vi "Keysight34461a.vi"(10 "Measurement Function (10: Voltage DC)":i32(ring)=10 items=["Continuity", "Current AC", "Current DC", "Diode", "Frequency", "Resistance 4-wire", "Period", "Resistance 2-wire", "Temperature", "Voltage AC", "Voltage DC", "Voltage DC Ratio", "Capacitance"], 11 "VISA resource name":refnum<visa-resource-name>) -> (3 "Display":string)   [LabVIEW 2024, in "Keysight_34461a.lvlib"]
doc: "This template is for the Queued Message Handler design pattern.\n\nThe Event Handling Loop generates messages based on user interface actions.\n\nThe Message Handling Loop processes messages generated by the Event Handling Loop, or by other messages. The messages are string values, so new messages can be added easily to the Message Cases case structure in the Message Handling Loop. Each message cluster can also provide an optional value for Message Data, which is a variant that can be converted to whatever message-specific data is required."
uses:
  Keysight_34461a.lvlib
  Settings/support/DMM_CONFIG.ctl
  controls/UI Data.ctl
  support/Message Queue/Enqueue Message (Single).vi
  <instrlib>/Agilent 3446X Series/Public/Data/Read (Single Point).vi
  <vilib>/Utility/error.llb/Error Cluster From Error Code.vi
  <vilib>/ErrorRing/Error Ring.xnode
  support/Message Queue/Message Queue.lvlib
  support/User Event - Stop/User Event - Stop.lvlib
  <instrlib>/Agilent 3446X Series/Agilent 3446X Series.lvlib
  Settings/Setting_Screen.lvlib
  Launcher/Launcher_DTU.lvlib
panel:
  in  "Read":bool
  in  "DMM_CONFIG":T1 {"CONFIG PARAMETER" items=["VOLTAGE", "CURRENT", "RESISTANCE", "POWER"]}
  in  "Config":string
  in  "DUT":string
  out "queue name 2":string
  out "queue name":string
  in  "Exit":bool
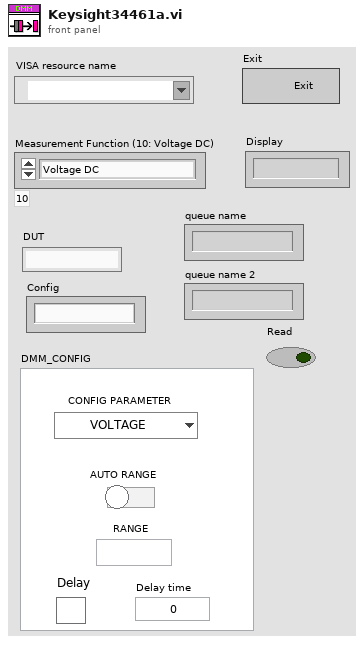
[diagram p1: front panel]
types:
  T1 = typedef "Setting_Screen.lvlib/DMM_CONFIG.ctl" = cluster{"CONFIG PARAMETER":u16, "AUTO RANGE":bool, "RANGE":string, "Delay":bool, "Delay time":dbl}
  T2 = typedef "Keysight_34461a.lvlib/UI Data.ctl" = cluster{"Boolean <Replace Me>":bool, "Display":string, "Numeric <Replace Me>":dbl, "Data Display Ref":refnum<vi>, "Exit Button Ref":refnum<vi>, "VISA resource name":refnum<visa-resource-name>, "notifier out":refnum<notifier>, "Config":string, "DUT":string, "Keysight_34461a_Q":refnum<queue>, "Config 2":string, "Count":u32}
  T3 = typedef "Keysight_34461a.lvlib/Message Queue.lvlib/All Message Queues.ctl" = cluster{"UI":refnum<queue>, "QSM":refnum<queue>}
  T4 = cluster{"Message":string, "Message Data":variant}
  T5 = enum16{"Read", "Write", "All_sections", "All_values", "Remove key&section"}
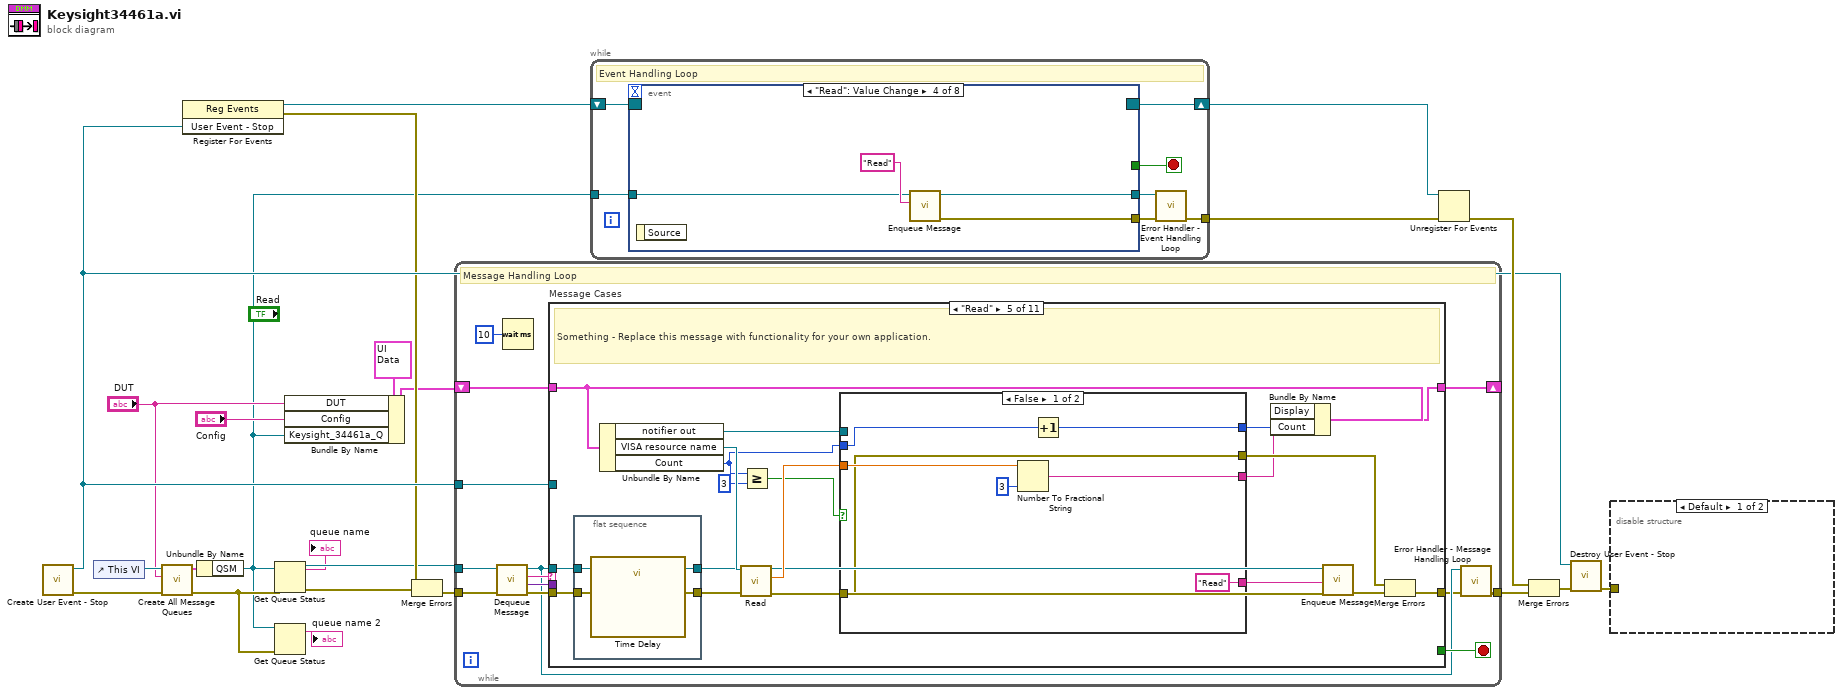
[diagram p0: block diagram]
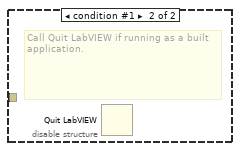
[diagram p2: hidden frame]
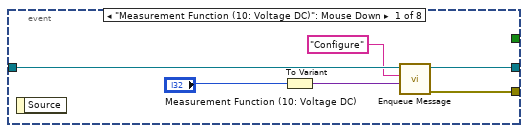
[diagram p3: hidden frame]
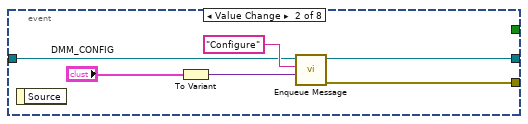
[diagram p4: hidden frame]
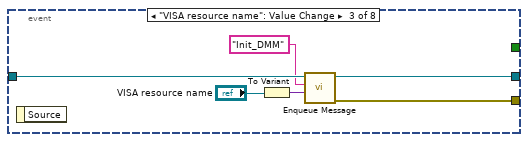
[diagram p5: hidden frame]
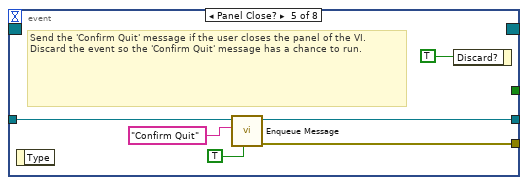
[diagram p6: hidden frame]
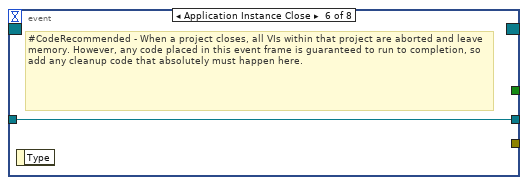
[diagram p7: hidden frame]
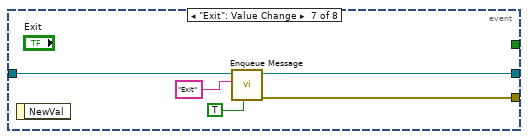
[diagram p8: hidden frame]
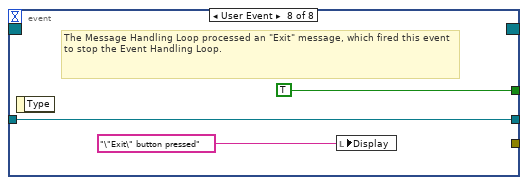
[diagram p9: hidden frame]
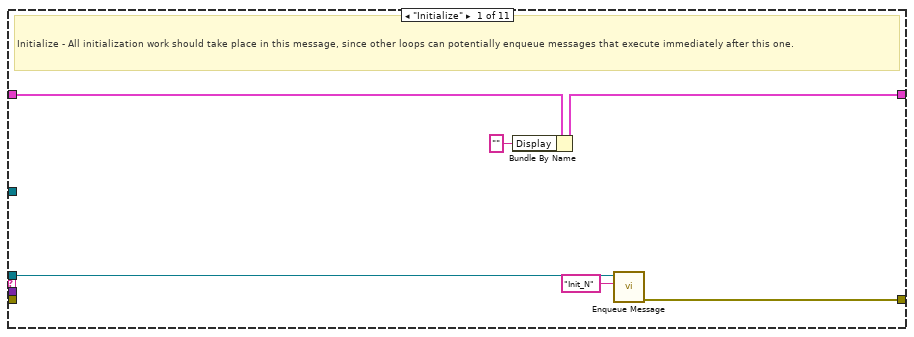
[diagram p10: hidden frame]
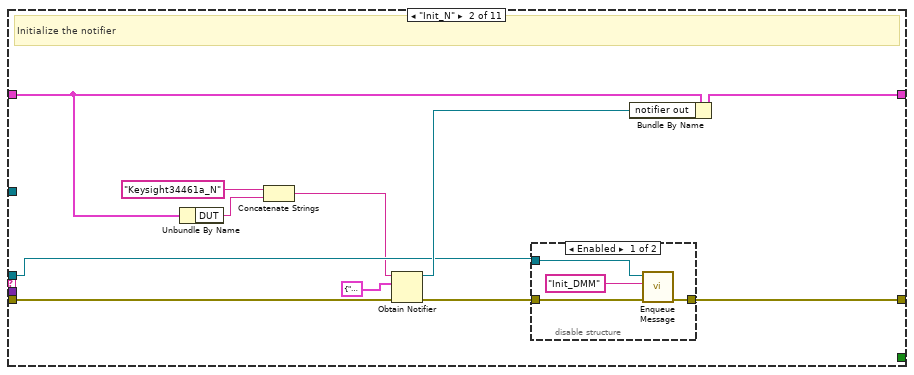
[diagram p11: hidden frame]
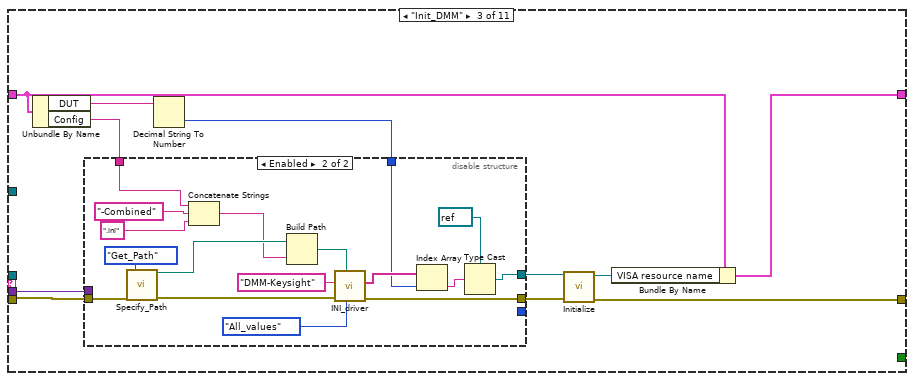
[diagram p13: hidden frame]
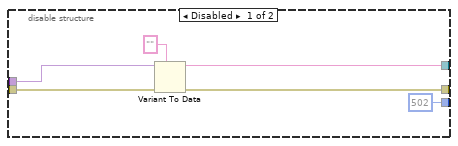
[diagram p14: hidden frame]
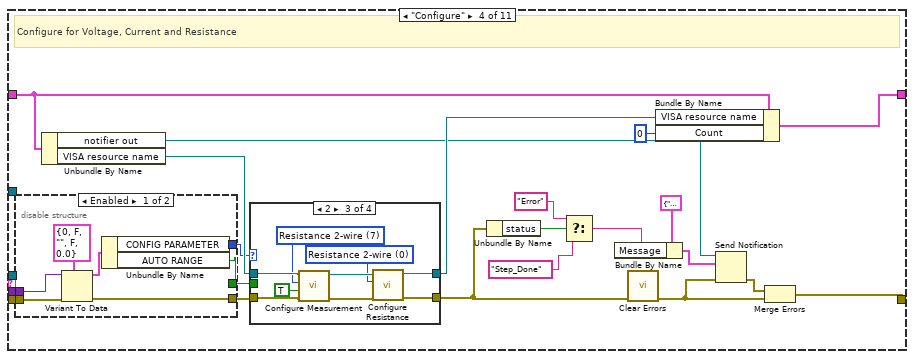
[diagram p15: hidden frame]
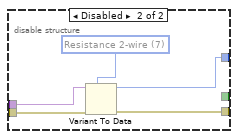
[diagram p16: hidden frame]
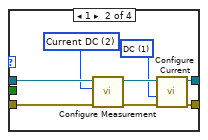
[diagram p18: hidden frame]
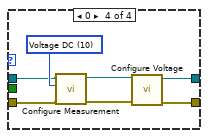
[diagram p19: hidden frame]
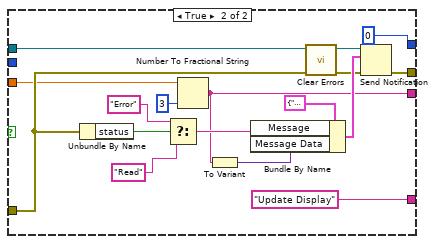
[diagram p20: hidden frame]
diagram:
  n1 = call "Create User Event - Stop.vi"() -> ("error out"=w21:errorcluster, "User Event - Stop"=w14:refnum<user-event>)  [unwired: 10 in]
  n2 = control-ref of="This VI"() -> (w5:refnum<vi>)
  n3 = call "Create All Message Queues.vi"("error in (no error)"=w21, "DUT"="DUT", "This VI"=w5) -> ("error out"=w8:errorcluster, "Message Queues out"=w23:T3)  [unwired: 7 in]
  n4 = register-events(w14) -> (reference out=w15:refnum<event-registration>, error out=w12:errorcluster)  [unwired: 2 in]
  n5 = Unbundle By Name(w23) -> ("QSM"=w1:refnum<queue>)
  n6 = Get Queue Status(queue=w1, error in (no error)=w8) -> (queue out=w10:refnum<queue>, queue name=→"queue name":string, error out=w11:errorcluster)  [unwired: 1 in, 5 out]
  n7 = Get Queue Status(queue=w1, error in (no error)=w8) -> (queue name=→"queue name 2":string)  [unwired: 1 in, 7 out]
  n8 = Bundle By Name(cluster=T2 {"Boolean <Replace Me>"=FALSE, "Display"="", "Numeric <Replace Me>"=0.0, "Data Display Ref"=refnum, "Exit Button Ref"=refnum, "VISA resource name"="", "notifier out"=refnum, "Config"="", "DUT"="", "Keysight_34461a_Q"=refnum, "Config 2"="", "Count"=0} ("Data Cluster"), "DUT"="DUT", "Config"="Config", "Keysight_34461a_Q"=w1) -> (w4:T2)
  n9 = Merge Errors(w12, w11) -> (w13:errorcluster)
  n10 = while {
    tunnel: w10 -> [w28]
    shift-right: [w35] -> _
    shift-left: w4 -> [w36]
    tunnel: w14 -> [w33]
    tunnel: w13 -> [w32]
    tunnel: [w26] -> w22
    stop <- w34 stop-if-true
    # "Message Handling Loop"
    n11 = call "Dequeue Message.vi"("error in (no error)"=w32, "Message Queue"=w28) -> ("error out"=w31:errorcluster, "Message Data"=w29:variant, "Message"=w30:string, "dup Message Queue"=w27:refnum<queue>)  [unwired: 6 in]
    n12 = Wait (ms)(milliseconds to wait=u32 10) -> ()  [unwired: 1 out]
    n13 = case "Message Cases" shown="\"Read\"" w30 {
      selector: w30 -> [_ _ _ _ _ _ _ _ _ _ w232]
      tunnel: w27 -> [w39 w46 _ _ w157 _ _ _ w215 w231 _]
      tunnel: w31 -> [_ w51 w65 w113 w159 w199 w205 w207 w210 w222 _]
      tunnel: [w42 w47 w69 w98 w165 w199 w200 w207 w216 w228 w233] -> w25
      tunnel: w36 -> [w41 w44 w62 w110 w167 w198 w204 w206 w212 w221 w234]
      tunnel: [w40 w50 w67 w107 w166 w198 w204 w206 w212 w221 w234] -> w35
      tunnel: [_ _ _ _ _ _ _ _ _ TRUE _] -> w34
      tunnel: w29 -> [_ _ w64 w112 _ _ w203 _ _ w223 _]
      tunnel: w33 -> [_ _ _ _ _ _ _ _ _ w227 _]
      frame "Initialize" {
        # "Initialize - All initialization work should take place in this message, since other loops can potentially enqueue messages that execute immediately after this one."
        n14 = Bundle By Name(cluster=w41, "Display"="") -> (w40:T2)
        n15 = call-poly "Enqueue Message.vi"("Message"="Init_N", "Message Queue"=w39) -> ("error out"=w42:errorcluster)  [unwired: 8 in, 1 out]
      }
      frame "Init_N" {
        # "Initialize the notifier"
        n16 = Unbundle By Name(w44) -> ("DUT"=w43:string)
        n17 = Concatenate Strings("Keysight34461a_N" ("String"), w43) -> (w45:string)
        n18 = Obtain Notifier(name (unnamed)=w45, notification data type=T4 {"Message"="", "Message Data"=variant} ("notification"), error in (no error)=w51) -> (notifier out=w49:refnum<notifier>, error out=w48:errorcluster)  [unwired: 1 in, 1 out]
        n19 = disable-structure shown="Enabled" {
          disable-tunnel: w48 -> [w56 w58]
          disable-tunnel: [w55 w58] -> w47
          disable-tunnel: w46 -> [w54 _]
          frame Enabled {
            n20 = call-poly "Enqueue Message.vi"("error in (no error)"=w56, "Message"="Init_DMM", "Message Queue"=w54) -> ("error out"=w55:errorcluster)  [unwired: 7 in, 1 out]
          }
          frame Disabled {
          }
        }
        n21 = Bundle By Name(cluster=w44, "notifier out"=w49) -> (w50:T2)
      }
      frame "Init_DMM" {
        n22 = Unbundle By Name(w62) -> ("DUT"=w60:string, "Config"=w63:string)
        n23 = Decimal String To Number(string=w60) -> (number=w59:i32)  [unwired: 2 in, 1 out]
        n24 = disable-structure shown="Enabled" {
          disable-tunnel: w65 -> [w75 w85]
          disable-tunnel: [w74 w84] -> w66
          disable-tunnel: w64 -> [w73 _]
          disable-tunnel: [w72 w79] -> w61
          disable-tunnel: [u16 502 _] -> _
          disable-tunnel: w63 -> [_ w80]
          disable-tunnel: w59 -> [_ w76]
          frame Disabled {
            n25 = Variant To Data(error in=w75, type="", Variant=w73) -> (data=w72:string, error out=w74:errorcluster)
          }
          frame Enabled {
            n26 = call "Specify_Path.vi"("Path_Enum"=enum16{"Find_Path", "Get_Path"}."Get_Path", "error in (no error)"=w85) -> ("Configurations"=w91:path, "error out"=w88:errorcluster)  [unwired: 6 in, 6 out]
            n27 = Concatenate Strings(w80, "-Combined" ("string"), ".ini" ("string")) -> (w81:string)
            n28 = Build Path(base path=w91, name or relative path=w81) -> (appended path=w90:path)
            n29 = call "INI_driver.vi"("Enum"=T5."All_values", "instrument file path"=w90, "error in (no error)"=w88, "Section"="DMM-Keysight") -> ("error out"=w84:errorcluster, "Values out"=w86:string[])  [unwired: 4 in, 2 out]
            n30 = Index Array(array=w86, index=w76) -> (element=w78:string)
            n31 = Type Cast(type=refnum<visa-resource-name> refnum ("VISA resource name 2"), x=w78) -> (*(type *) &x=w79:refnum<visa-resource-name>)
          }
        }
        n32 = call <instrlib>:"Initialize.vi"("error in (no error)"=w66, "VISA resource name"=w61) -> ("error out"=w69:errorcluster, "VISA resource name out"=w68:refnum<visa-resource-name>)  [unwired: 8 in]
        n33 = Bundle By Name(cluster=w62, "VISA resource name"=w68) -> (w67:T2)
      }
      frame "Configure" {
        # "Configure for Voltage, Current and Resistance"
        n34 = disable-structure shown="Enabled" {
          disable-tunnel: w113 -> [w120 w125]
          disable-tunnel: w112 -> [w119 w122]
          disable-tunnel: [w118 w124] -> w111
          disable-tunnel: [w116 w121] -> w108
          disable-tunnel: [w114 _] -> w94
          frame Enabled {
            n35 = Variant To Data(error in=w120, type=T1 {"CONFIG PARAMETER"=0, "AUTO RANGE"=FALSE, "RANGE"="", "Delay"=FALSE, "Delay time"=0.0} ("DMM_CONFIG"), Variant=w119) -> (data=w115:T1, error out=w118:errorcluster)
            n36 = Unbundle By Name(w115) -> ("CONFIG PARAMETER"=w116:u16, "AUTO RANGE"=w114:bool)
          }
          frame Disabled {
            w123 = 7 items=["Continuity", "Current AC", "Current DC", "Diode", "Frequency", "Resistance 4-wire", "Period", "Resistance 2-wire", "Temperature", "Voltage AC", "Voltage DC", "Voltage DC Ratio", "Capacitance"] ("Measurement Function (10: Voltage DC)")
            n37 = Variant To Data(error in=w125, type=w123, Variant=w122) -> (data=w121:i32, error out=w124:errorcluster)
          }
        }
        n38 = Unbundle By Name(w110) -> ("notifier out"=w100:refnum<notifier>, "VISA resource name"=w109:refnum<visa-resource-name>)
        n39 = case shown="2" w108 {
          tunnel: w111 -> [w127 w133 w142 w146]
          tunnel: [w127 w135 w144 w151] -> w97
          tunnel: w109 -> [w126 w132 w140 w148]
          tunnel: [w126 w134 w143 w150] -> w106
          tunnel: w94 -> [_ _ _ _]
          frame Default {
          }
          frame 1 {
            w128 = 1 items=["AC", "DC"] ("Current Type (0: AC)")
            w129 = 2 items=["Continuity", "Current AC", "Current DC", "Diode", "Frequency", "Resistance 4-wire", "Period", "Resistance 2-wire", "Temperature", "Voltage AC", "Voltage DC", "Voltage DC Ratio", "Capacitance"] ("Measurement Function (10: Voltage DC)")
            n40 = call <instrlib>:"Configure Measurement.vi"("error in (no error)"=w133, "Measurement Function (10: Voltage DC)"=w129, "VISA resource name"=w132) -> ("error out"=w131:errorcluster, "VISA resource name out"=w130:refnum<visa-resource-name>)  [unwired: 7 in]
            n41 = call <instrlib>:"Configure Current.vi"("error in (no error)"=w131, "Current Type (0: AC)"=w128, "VISA resource name"=w130) -> ("error out"=w135:errorcluster, "VISA resource name out"=w134:refnum<visa-resource-name>)  [unwired: 7 in]
          }
          frame 2 {
            w137 = 0 items=["Resistance 2-wire", "Resistance 4-wire"] ("Resistance Type (0: Resistance 2-wire)")
            w138 = 7 items=["Continuity", "Current AC", "Current DC", "Diode", "Frequency", "Resistance 4-wire", "Period", "Resistance 2-wire", "Temperature", "Voltage AC", "Voltage DC", "Voltage DC Ratio", "Capacitance"] ("Measurement Function (10: Voltage DC)")
            n42 = call <instrlib>:"Configure Measurement.vi"("error in (no error)"=w142, "Auto Range (T: Enable)"=TRUE, "Measurement Function (10: Voltage DC)"=w138, "VISA resource name"=w140) -> ("error out"=w141:errorcluster, "VISA resource name out"=w139:refnum<visa-resource-name>)  [unwired: 6 in]
            n43 = call <instrlib>:"Configure Resistance.vi"("error in (no error)"=w141, "Resistance Type (0: Resistance 2-wire)"=w137, "VISA resource name"=w139) -> ("error out"=w144:errorcluster, "VISA resource name out"=w143:refnum<visa-resource-name>)  [unwired: 7 in]
          }
          frame 0 {
            w149 = 10 items=["Continuity", "Current AC", "Current DC", "Diode", "Frequency", "Resistance 4-wire", "Period", "Resistance 2-wire", "Temperature", "Voltage AC", "Voltage DC", "Voltage DC Ratio", "Capacitance"] ("Measurement Function (10: Voltage DC)")
            n44 = call <instrlib>:"Configure Measurement.vi"("error in (no error)"=w146, "Measurement Function (10: Voltage DC)"=w149, "VISA resource name"=w148) -> ("error out"=w145:errorcluster, "VISA resource name out"=w147:refnum<visa-resource-name>)  [unwired: 7 in]
            n45 = call <instrlib>:"Configure Voltage.vi"("error in (no error)"=w145, "VISA resource name"=w147) -> ("error out"=w151:errorcluster, "VISA resource name out"=w150:refnum<visa-resource-name>)  [unwired: 8 in]
          }
        }
        n46 = Unbundle By Name(w97) -> ("status"=w105:bool)
        n47 = Select(t="Error" ("f"), s=w105, f="Step_Done" ("Message")) -> (s? t:f=w102:string)
        n48 = Bundle By Name(cluster=T4 {"Message"="", "Message Data"=variant} ("notification"), "Message"=w102) -> (w101:T4)
        n49 = call <vilib>:"Clear Errors.vi"("error in (no error)"=w97) -> ("error out"=w95:errorcluster)  [unwired: 5 in, 1 out]
        n50 = Bundle By Name(cluster=w110, "VISA resource name"=w106, "Count"=u32 0) -> (w107:T2)
        n51 = Send Notification(notification=w101, notifier=w100, error in (no error)=w95) -> (error out=w96:errorcluster)  [unwired: 1 out]
        n52 = Merge Errors(w96, w95) -> (w98:errorcluster)
      }
      frame "Read" {
        # "Something - Replace this message with functionality for your own application."
        n53 = flat-sequence {
          tunnel: w159 -> [w196]
          tunnel: [w194] -> w158
          tunnel: w157 -> [w195]
          tunnel: [w195] -> w156
          frame #0 {
            n54 = call "Time Delay"("error in (no error)"=w196) -> ("error out"=w194:errorcluster)  [unwired: 10 in]
          }
        }
        n55 = Unbundle By Name(w167) -> ("notifier out"=w163:refnum<notifier>, "VISA resource name"=w168:refnum<visa-resource-name>, "Count"=w152:u32)
        n56 = call-poly <instrlib>:"Read.vi"("error in (no error)"=w158, "VISA resource name"=w168) -> ("error out"=w162:errorcluster, "Measurement"=w161:dbl)  [unwired: 7 in, 1 out]
        n57 = Greater Or Equal?(x=w152, y=u32 3) -> (x >= y?=w154:bool)
        n58 = case shown="False" w154 {
          tunnel: ["Read" ("Message") "Update Display" ("Message")] -> w169
          tunnel: [w173 w186] -> w164
          tunnel: w163 -> [_ w185]
          tunnel: w162 -> [w173 w184]
          tunnel: w161 -> [w176 w182]
          tunnel: [w174 w180] -> w160
          tunnel: [w171 u32 0 ("Count")] -> w153
          tunnel: w152 -> [w172 _]
          frame False {
            n59 = Number To Fractional String(number=w176, precision (6)=i16 3) -> (F-format string=w174:string)  [unwired: 2 in]
            n60 = Increment(x=w172) -> (x+1=w171:u32)
          }
          frame True {
            n61 = Unbundle By Name(w184) -> ("status"=w192:bool)
            n62 = Select(t="Error" ("f"), s=w192, f="Read" ("Message")) -> (s? t:f=w188:string)
            n63 = Number To Fractional String(number=w182, precision (6)=i16 3) -> (F-format string=w180:string)  [unwired: 2 in]
            n64 = To Variant(anything=w180) -> (Variant=w181:variant)
            n65 = Bundle By Name(cluster=T4 {"Message"="", "Message Data"=variant} ("notification"), "Message"=w188, "Message Data"=w181) -> (w187:T4)
            n66 = call <vilib>:"Clear Errors.vi"("error in (no error)"=w184) -> ("error out"=w183:errorcluster)  [unwired: 5 in, 1 out]
            n67 = Send Notification(notification=w187, notifier=w185, error in (no error)=w183) -> (error out=w186:errorcluster)  [unwired: 1 out]
          }
        }
        n68 = Bundle By Name(cluster=w167, "Display"=w160, "Count"=w153) -> (w166:T2)
        n69 = call-poly "Enqueue Message.vi"("error in (no error)"=w162, "Message"=w169, "Message Queue"=w156) -> ("error out"=w170:errorcluster)  [unwired: 7 in, 1 out]
        n70 = Merge Errors(w164, w170) -> (w165:errorcluster)
      }
      frame "Update Display" {
        # "Update Display - Convert the message data to a string to display in the Data Display indicator."
        n71 = Unbundle By Name(w198) -> ("Display"=→"Display":string)
      }
      frame "Error" {
        # "Error - Display an error dialog. This message is sent by the \"Error Handler\" VIs at the end of other loops in this application."
        n72 = Variant To Data(error in=w205, type=errorcluster {"status"=FALSE, "code"=0, "source"=""} ("error constant"), Variant=w203) -> (data=w201:errorcluster, error out=w200:errorcluster)
        n73 = call <vilib>:"Simple Error Handler.vi"("error in (no error)"=w201) -> ()  [unwired: 4 in, 5 out]
      }
      frame "Reset" {
      }
      frame "Confirm Quit" {
        # "Confirm Quit - Message that can confirm whether or not the user wants to exit the application."
        n74 = Unbundle By Name(w212) -> ("notifier out"=w211:refnum<notifier>)
        n75 = Release Notifier(notifier=w211, force destroy? (F)=TRUE, error in (no error)=w210) -> (error out=w209:errorcluster)  [unwired: 2 out]
        n76 = call-poly "Enqueue Message.vi"("Priority Message? (F)"=TRUE, "error in (no error)"=w209, "Message"="Exit", "Message Queue"=w215) -> ("error out"=w216:errorcluster)  [unwired: 6 in, 1 out]
      }
      frame "Exit" {
        # "Stop the VI"
        # "Release the message queue reference"
        # "Exit - Exit the application."
        n77 = Unbundle By Name(w221) -> ("VISA resource name"=w220:refnum<visa-resource-name>)
        n78 = Variant To Data(type=errorcluster {"status"=FALSE, "code"=0, "source"=""} ("error constant"), Variant=w223) -> (data=w224:errorcluster)  [unwired: 1 in, 1 out]
        n79 = call <vilib>:"Simple Error Handler.vi"("error in (no error)"=w224) -> ()  [unwired: 4 in, 5 out]
        n80 = call <instrlib>:"Close.vi"("error in (no error)"=w222, "VISA resource name"=w220) -> ("error out"=w218:errorcluster)  [unwired: 9 in]
        n81 = call "Fire User Event - Stop.vi"("User Event - Stop"=w227) -> ("error out"=w226:errorcluster)  [unwired: 10 in]
        n82 = call <vilib>:"Clear Errors.vi"("error in (no error)"=w218) -> ("error out"=w217:errorcluster)  [unwired: 5 in, 1 out]
        n83 = call <vilib>:"Clear Errors.vi"("error in (no error)"=w226) -> ("error out"=w219:errorcluster)  [unwired: 5 in, 1 out]
        n84 = Release Queue(queue=w231, error in (no error)=w217) -> (error out=w229:errorcluster)  [unwired: 1 in, 2 out]
        n85 = Merge Errors(w219, w229) -> (w228:errorcluster)
      }
      frame Default {
        # "'Default' case only runs if there is a message that isn't defined in any of the other cases.  Output a programming error."
        n86 = xnode "Error Ring"("parameter 0"=w232) -> ("error out"=w233:errorcluster)
      }
    }
    n87 = call "Error Handler - Message Handling Loop.vi"("error in (no error)"=w25, "Message Queue"=w27) -> ("dup error in"=w26:errorcluster)  [unwired: 8 in, 1 out]
  }
  n88 = while {
    tunnel: w1 -> [w248]
    shift-right: [w246] -> w18
    shift-left: w15 -> [w247]
    tunnel: [w242] -> w16
    stop <- w244 stop-if-true
    # "Event Handling Loop"
    n89 = event shown="[3] \"Read\": Value Change" {
      selector: w247 -> [_ _ _ _ _ _ _ _]
      dyn-events: [_ _ _ _ _ _ _ _] -> w246
      timeout: _ -> [_ _ _ _ _ _ _ _]
      tunnel: [_ _ _ _ _ _ _ TRUE ("Discard?")] -> w244
      tunnel: w248 -> [w254 w258 w262 w269 w275 w277 w282 w285]
      tunnel: [w251 w256 w266 w268 w274 _ w281 _] -> w245
      tunnel: [w253 w257 w263 w267 w273 w277 w280 w285] -> w243
      event "Measurement Function (10: Voltage DC)": Mouse Down {
        n90 = event-data() -> ()  [unwired: 1 in, 1 out]
        n91 = To Variant(anything="Measurement Function (10: Voltage DC)") -> (Variant=w249:variant)
        n92 = call-poly "Enqueue Message.vi"("Message Data"=w249, "Message"="Configure", "Message Queue"=w254) -> ("error out"=w251:errorcluster, "dup Message Queue"=w253:refnum<queue>)  [unwired: 7 in]
      }
      event Value Change {
        n93 = event-data() -> ()  [unwired: 1 in, 1 out]
        n94 = To Variant(anything="DMM_CONFIG") -> (Variant=w259:variant)
        n95 = call-poly "Enqueue Message.vi"("Message Data"=w259, "Message"="Configure", "Message Queue"=w258) -> ("error out"=w256:errorcluster, "dup Message Queue"=w257:refnum<queue>)  [unwired: 7 in]
      }
      event "VISA resource name": Value Change {
        n96 = event-data() -> ()  [unwired: 1 in, 1 out]
        n97 = To Variant(anything="VISA resource name") -> (Variant=w264:variant)
        n98 = call-poly "Enqueue Message.vi"("Message Data"=w264, "Message"="Init_DMM", "Message Queue"=w262) -> ("error out"=w266:errorcluster, "dup Message Queue"=w263:refnum<queue>)  [unwired: 7 in]
      }
      event "Read": Value Change {
        n99 = event-data() -> ()  [unwired: 1 in, 1 out]
        n100 = call-poly "Enqueue Message.vi"("Message"="Read", "Message Queue"=w269) -> ("error out"=w268:errorcluster, "dup Message Queue"=w267:refnum<queue>)  [unwired: 8 in]
      }
      event Panel Close? {
        # "Send the 'Confirm Quit' message if the user closes the panel of the VI. Discard the event so the 'Confirm Quit' message has a chance to run."
        n101 = event-data() -> ()  [unwired: 1 in, 1 out]
        n102 = call-poly "Enqueue Message.vi"("Priority Message? (F)"=TRUE, "Message"="Confirm Quit", "Message Queue"=w275) -> ("error out"=w274:errorcluster, "dup Message Queue"=w273:refnum<queue>)  [unwired: 7 in]
        n103 = event-data("Discard?"=TRUE) -> ()  [unwired: 1 in, 1 out]
      }
      event Application Instance Close {
        # "#CodeRecommended - When a project closes, all VIs within that project are aborted and leave memory. However, any code placed in this event frame is guaranteed to run to completion, so add any cleanup code that absolutely must happen here."
        n104 = event-data() -> ()  [unwired: 1 in, 1 out]
      }
      event "Exit": Value Change {
        n105 = event-data() -> ()  [unwired: 1 in, 1 out]
        n106 = call-poly "Enqueue Message.vi"("Priority Message? (F)"=TRUE, "Message"="Exit", "Message Queue"=w282) -> ("error out"=w281:errorcluster, "dup Message Queue"=w280:refnum<queue>)  [unwired: 7 in]
      }
      event User Event {
        # "The Message Handling Loop processed an \"Exit\" message, which fired this event to stop the Event Handling Loop."
        n107 = event-data() -> ()  [unwired: 1 in, 1 out]
        n108 = local write "Display"("\"Exit\" button pressed" ("VI Stopped")) -> ()
      }
    }
    n109 = call "Error Handler - Event Handling Loop.vi"("error in (no error)"=w245, "Message Queue"=w243) -> ("dup error in"=w242:errorcluster)  [unwired: 8 in, 1 out]
  }
  n110 = Unregister For Events(event registration refnum=w18, error in=w16) -> (error out=w19:errorcluster)
  n111 = Merge Errors(w19, w22) -> (w20:errorcluster)
  n112 = call "Destroy User Event - Stop.vi"("error in (no error)"=w20, "User Event - Stop"=w14) -> ("error out"=w17:errorcluster)  [unwired: 9 in]
  n113 = disable-structure shown="Default" {
    disable-tunnel: w17 -> [_ _]
    frame condition #0 (active) {
    }
    frame condition #1 {
      # "Call Quit LabVIEW if running as a built application."
      n114 = Quit LabVIEW() -> ()  [unwired: 1 in]
    }
  }
